vi "JSON Value.vi"(8 "error in (no error)":errorcluster, 10 "Start Index":i32, 11 "JSON":string="[{\"Name\": \"as\\\\\\\"d\\\\[f\",\"Mode\": 1,\"# Pulses\": 0,\"delta\": 0.000000,\"Start BDP\": 0.000000,\"End BDP\": 0.000000,\"Start E\": 0.000000,\"End E\": 0.000000,\"Start Angle\": 0.000000,\"End Angle\": 0.000000,\"Motor wait\": true,\"Motor velocity\": 0.000000,\"Iterations\": 0.000000,\"Interval\": 0.000000,\"ExtTriggerDelay\": 0.000000}]") -> (0 "error out":errorcluster, 2 "End Index":u32, 3 "Value":variant)   [LabVIEW 2011]
panel:
  out "End Index 2":u32
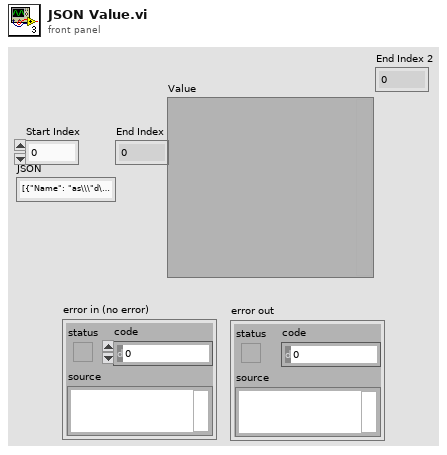
[diagram p1: front panel]
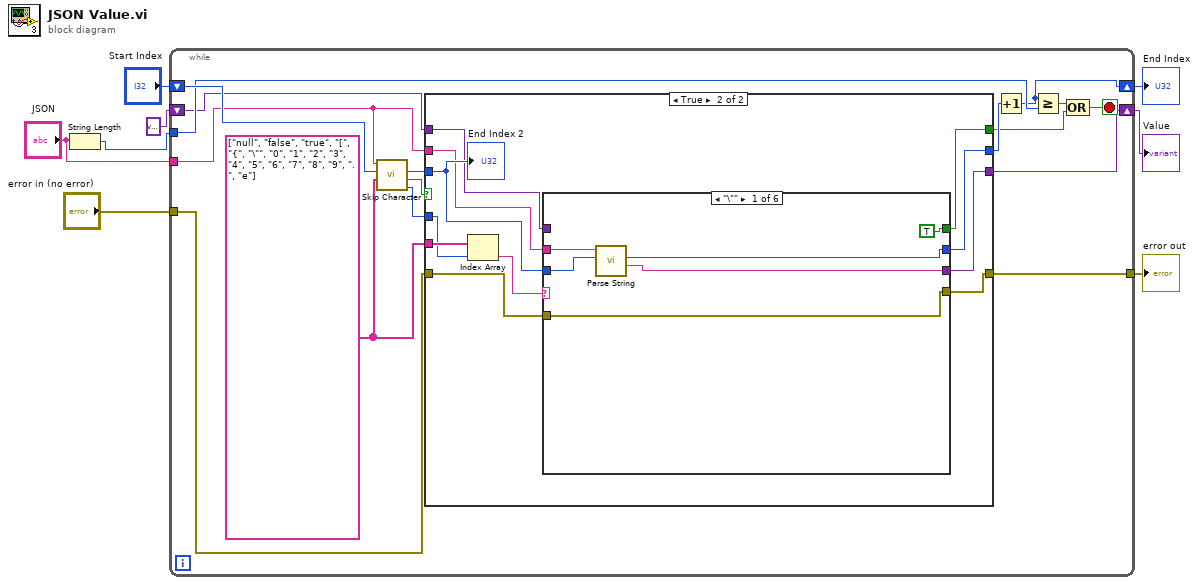
[diagram p0: block diagram]
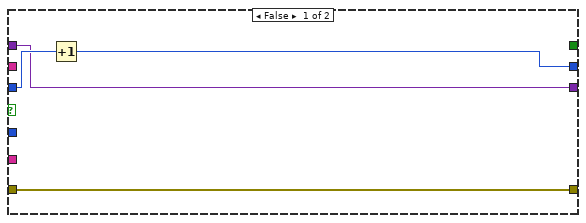
[diagram p2: hidden frame]
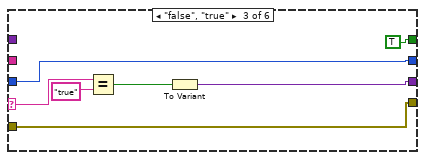
[diagram p4: hidden frame]
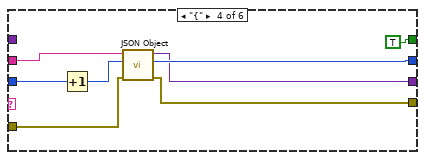
[diagram p5: hidden frame]
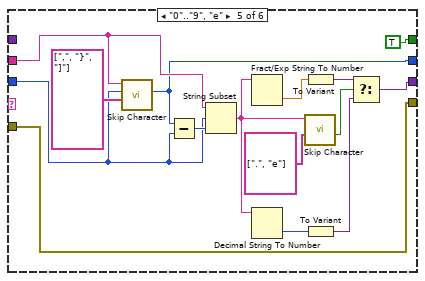
[diagram p6: hidden frame]
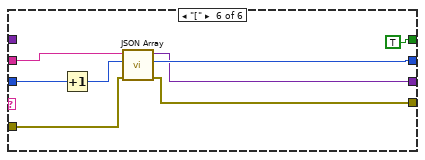
[diagram p7: hidden frame]
diagram:
  n1 = String Length(string="JSON") -> (length=w3:i32)
  n2 = while {
    tunnel: "JSON" -> [w17]
    shift-right: [w14] -> w5
    shift-left: "Start Index" -> [w24]
    tunnel: w3 -> [w18]
    shift-right: [w16] -> w8
    shift-left: variant ("Variant") -> [w15]
    tunnel: "error in (no error)" -> [w10]
    tunnel: [w9] -> w1
    stop <- w11 stop-if-true
    w21 = string[] ["null", "false", "true", "[", "{", "\"", "0", "1", "2", "3", "4", "5", "6", "7", "8", "9", ".", "e"] ("string array")
    n3 = call "Skip Character.vi"("Stop Strings"=w21, "Start Index"=w24, "JSON"=w17) -> ("Found String Index"=w22:i32, "Found Stop Character"=w23:bool, "End Index"=w20:u32)  [unwired: 6 in]
    n4 = case shown="True" w23 {
      tunnel: w22 -> [_ w38]
      tunnel: w21 -> [_ w39]
      tunnel: w20 -> [w28 w36]
      tunnel: [w27 w35] -> w19
      tunnel: w17 -> [_ w34]
      tunnel: [w26 w33] -> w16
      tunnel: w15 -> [w26 w32]
      tunnel: [_ w31] -> w12
      tunnel: w10 -> [w25 w30]
      tunnel: [w25 w29] -> w9
      frame False {
        n5 = Increment(x=w28) -> (x+1=w27:u32)
      }
      frame True {
        n6 = Index Array(array=w39, index=w38) -> (element=w37:string)
        n7 = case shown="\"\\\"\"" w37 {
          selector: w37 -> [_ _ w54 _ _ _]
          tunnel: w36 -> [w42 w47 w55 w62 w73 w86]
          tunnel: [w44 w47 w55 w61 w74 w85] -> w35
          tunnel: w34 -> [w45 _ _ w63 w76 w84]
          tunnel: [w41 w48 w51 w59 w65 w82] -> w33
          tunnel: w32 -> [_ w48 _ _ _ _]
          tunnel: [TRUE _ TRUE TRUE TRUE TRUE] -> w31
          tunnel: w30 -> [w40 w46 w49 w57 w64 w80]
          tunnel: [w40 w46 w49 w56 w64 w79] -> w29
          frame "\"" {
            n8 = call "Parse String.vi"("Start Index"=w42, "JSON"=w45) -> ("String"=w41:string, "EndIndex"=w44:i32)  [unwired: 6 in, 1 out]
          }
          frame Default {
          }
          frame "false", "true" {
            n9 = Equal?(x=w54, y="true") -> (x = y?=w52:bool)
            n10 = To Variant(anything=w52) -> (Variant=w51:variant)
          }
          frame "{" {
            n11 = Increment(x=w62) -> (x+1=w60:u32)
            n12 = call "JSON Object.vi"("error in (no error)"=w57, "Start Index"=w60, "JSON"=w63) -> ("error out"=w56:errorcluster, "End Index"=w61:i32, "VCluster"=w59:variant)  [unwired: 6 in]
          }
          frame "0".."9", "e" {
            n13 = call "Skip Character.vi"("Stop Strings"=string[] [",", "}", "]"], "Start Index"=w73, "JSON"=w76) -> ("End Index"=w74:u32)  [unwired: 6 in, 2 out]
            n14 = Subtract(x=w74, y=w73) -> (x-y=w75:u32)
            n15 = String Subset(string=w76, offset (0)=w73, length (rest)=w75) -> (substring=w72:string)
            n16 = Fract/Exp String To Number(string=w72) -> (number=w70:dbl)  [unwired: 3 in, 1 out]
            n17 = Decimal String To Number(string=w72) -> (number=w69:i32)  [unwired: 2 in, 1 out]
            n18 = call "Skip Character.vi"("Stop Strings"=string[] [".", "e"], "JSON"=w72) -> ("Found Stop Character"=w68:bool)  [unwired: 7 in, 2 out]
            n19 = To Variant(anything=w70) -> (Variant=w67:variant)
            n20 = To Variant(anything=w69) -> (Variant=w66:variant)
            n21 = Select(t=w67, s=w68, f=w66) -> (s? t:f=w65:variant)
          }
          frame "[" {
            n22 = Increment(x=w86) -> (x+1=w83:u32)
            n23 = call "JSON Array.vi"("error in (no error)"=w80, "Start Index"=w83, "JSON"=w84) -> ("error out"=w79:errorcluster, "End Index"=w85:i32, "VArray"=w82:variant)  [unwired: 6 in]
          }
        }
        "End Index 2" <- w36
      }
    }
    n24 = Increment(x=w19) -> (x+1=w14:u32)
    n25 = Greater Or Equal?(x=w14, y=w18) -> (x >= y?=w13:bool)
    n26 = Compound Arithmetic op=OR(w13, w12) -> (w11:bool)
  }
  "Value" <- w8
  "End Index" <- w5
  "error out" <- w1
